vi "Diff Timer.vi"(8 "error in (no error)":errorcluster) -> (0 "error out":errorcluster, 3 "time diff(s)":dbl)   [LabVIEW 2020]
doc: "Detects the time difference of each cycle of VI operation."
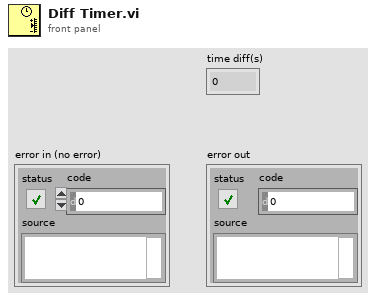
[diagram p1: front panel]
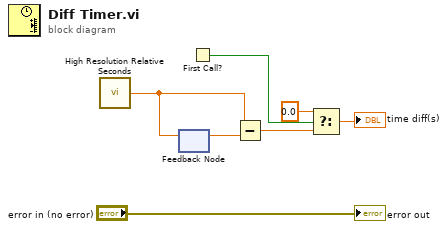
[diagram p0: block diagram]
diagram:
  n1 = call <vilib>:"High Resolution Relative Seconds.vi"() -> ("relative seconds"=w7:dbl)
  n2 = feedback-in #1(w7) -> ()
  n3 = feedback #1() -> (w6:dbl)  [unwired: 1 in]
  n4 = First Call?() -> (First Call?: T/F=w4:bool)
  n5 = Subtract(x=w7, y=w6) -> (x-y=w3:dbl)
  n6 = Select(t=0.0, s=w4, f=w3) -> (s? t:f=→"time diff(s)":dbl)
  "error out" <- "error in (no error)"
